vi "load data_backup.vi"(7 "Append dataset":bool, 10 "existing file numbers":string[](array[string]), 11 "existing data cluster":cluster{"array type (2D Dbl)":dbl[][]}[](array[cluster])) -> (2 "data names":string[](array[string]), 3 "data cluster":cluster{"all data":dbl[][]}[](array[cluster]))   [LabVIEW 2020]
uses:
  <vilib>/Utility/file.llb/Read Delimited Spreadsheet (DBL).vi
panel:
  in  "Done":bool
  out "# of importe files":i32
  in  "numbered file":T1={"FILE HEADER"="20120217", "FROM"="012", "TO"="012", "Excluding\nFrom"="", "Excluding\nTo"="", "Start Loading\ndata files"=FALSE, "cancel"=FALSE}
  in  "Cancel button":bool
  in  "Import Menu":T2(ring)
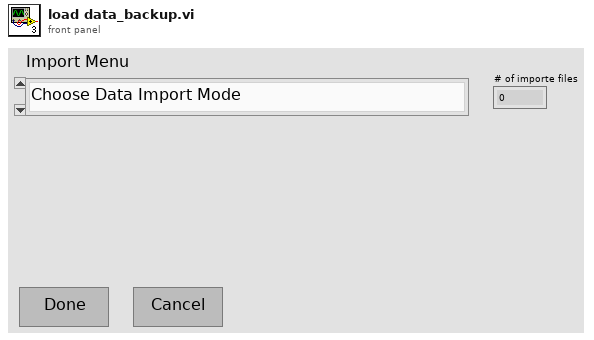
[diagram p1: front panel]
types:
  T1 = cluster{"FILE HEADER":string, "FROM":string, "TO":string, "Excluding\nFrom":string, "Excluding\nTo":string, "Start Loading\ndata files":bool, "cancel":bool}
  T2 = enum16{"Choose Data Import Mode", "Numbered NML Data Acq files saved in the drive", "Import current data being taken", "Manual selection of text file(s) ", "Manual Input of single XY plot(s)", "Manual Input of a worksheet"}
  T3 = enum16{"Choose Data Import Mode", "Numbered NML Data Acq files saved in the drive", "Import current NML Data Acq being taken", "Manual selection of text file(s) ", "Manual Input of XY arrays", "Manual Input of a worksheet"}
  T4 = enum16{"Left Button", "Center Button", "Right Button", "Window Close"}
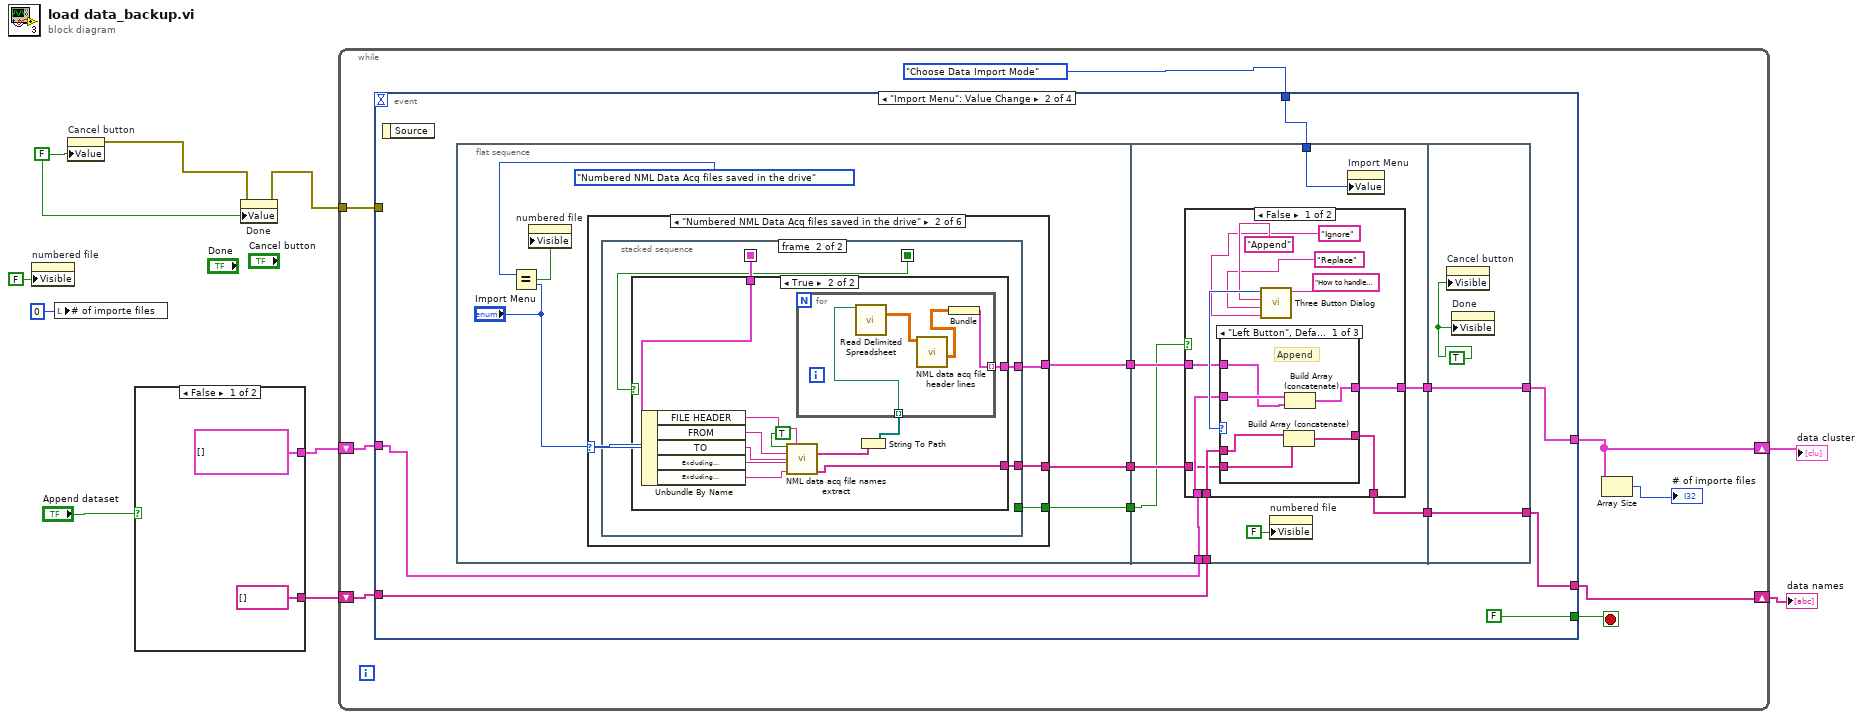
[diagram p0: block diagram]
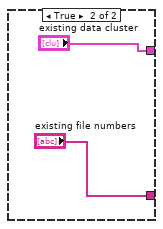
[diagram p2: hidden frame]
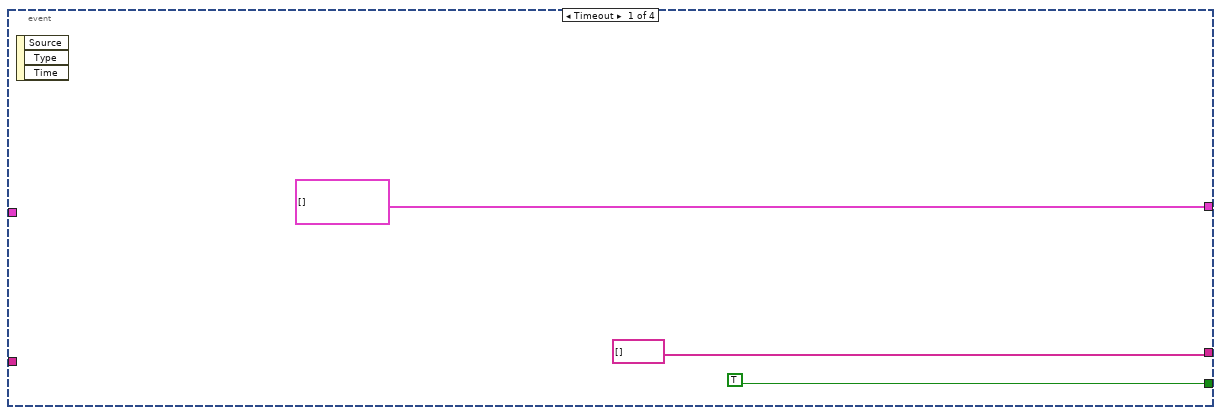
[diagram p3: hidden frame]
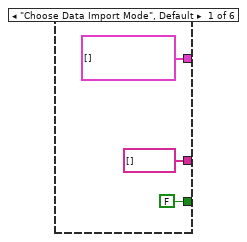
[diagram p4: hidden frame]
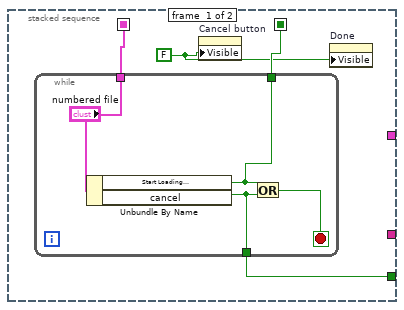
[diagram p5: hidden frame]
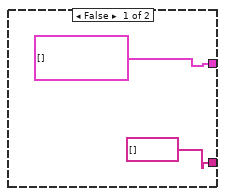
[diagram p6: hidden frame]
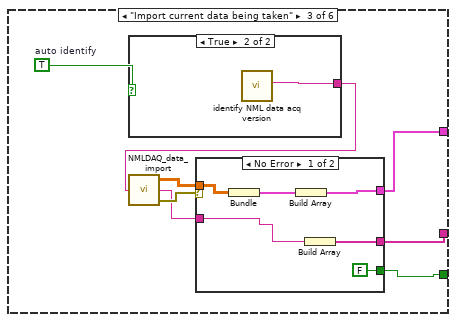
[diagram p7: hidden frame]
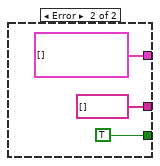
[diagram p8: hidden frame]
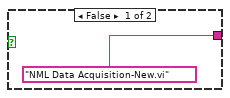
[diagram p9: hidden frame]
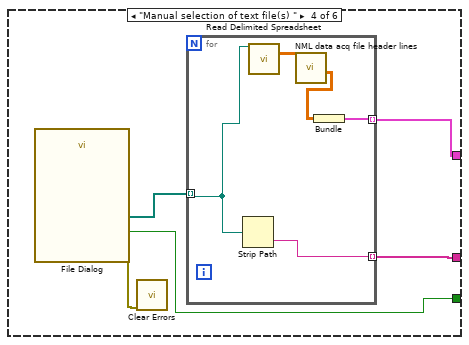
[diagram p10: hidden frame]
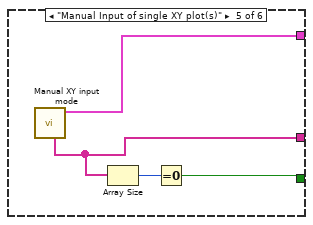
[diagram p11: hidden frame]
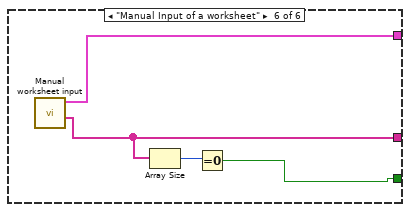
[diagram p12: hidden frame]
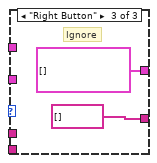
[diagram p14: hidden frame]
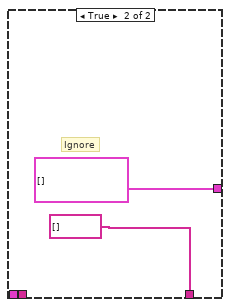
[diagram p15: hidden frame]
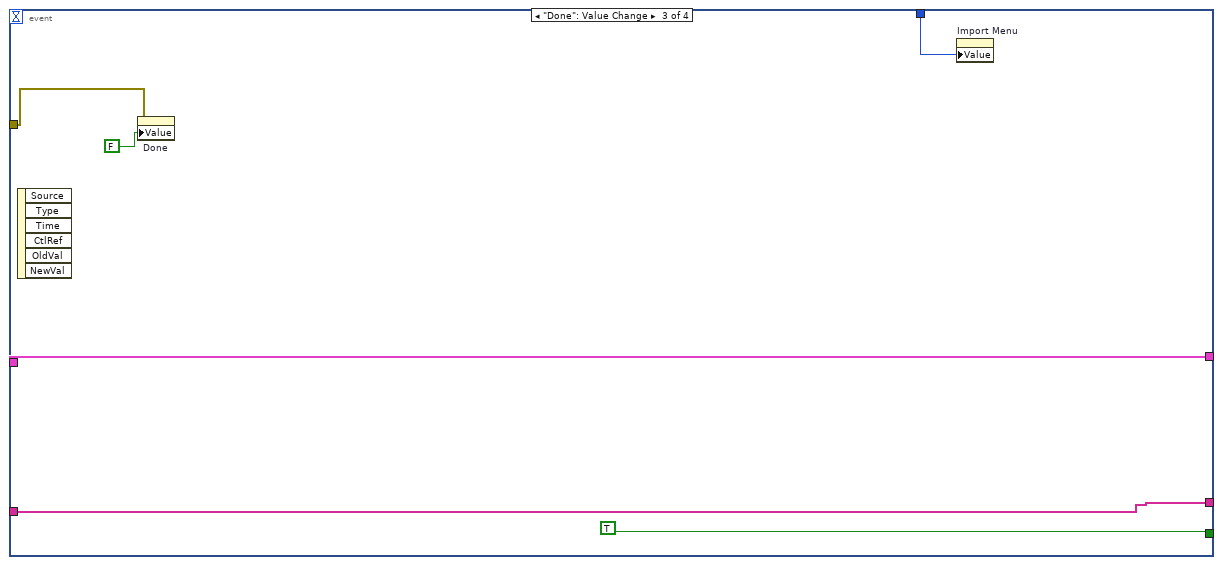
[diagram p16: hidden frame]
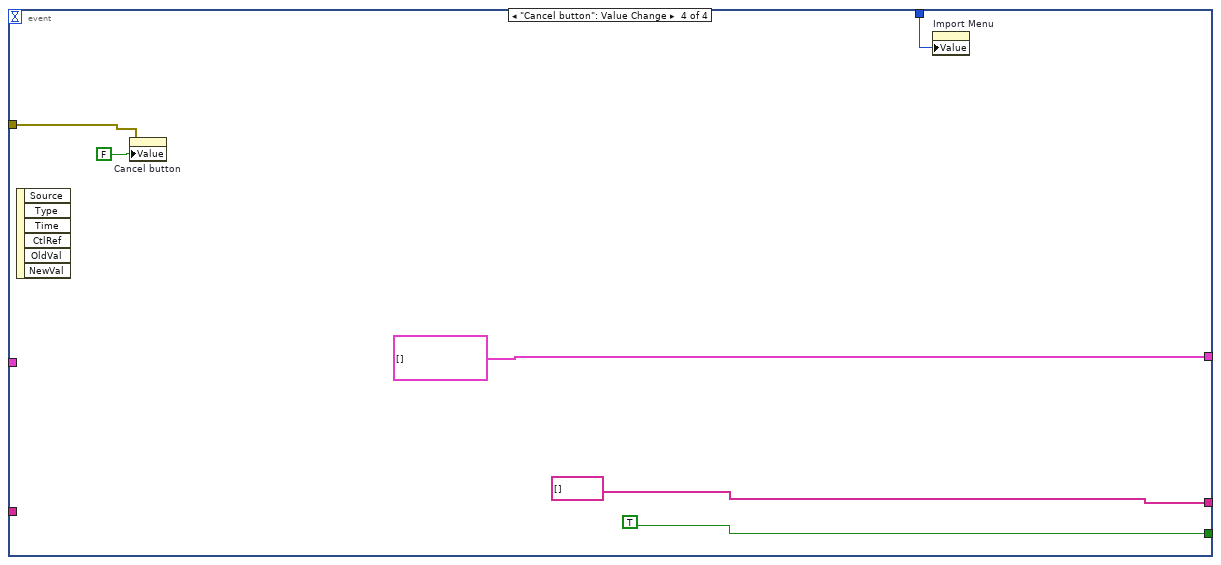
[diagram p17: hidden frame]
diagram:
  w2 = FALSE ("Value (Signaling)")
  n1 = property on="numbered file" class="Clust"("Visible"=FALSE) -> ()  [unwired: 2 in, 2 out]
  n2 = local write "# of importe files"(0 ("# of data files")) -> ()
  n3 = property on="Cancel button" class="Bool (strict)"("Value"=w2) -> (error out=w3:errorcluster)  [unwired: 2 in, 1 out]
  n4 = case shown="False" "Append dataset" {
    tunnel: [cluster{"array type (2D Dbl)":dbl[][]}[] [] ("existing data cluster") "existing data cluster"] -> w6
    tunnel: [string[] [] ("existing file numbers") "existing file numbers"] -> w5
    frame False {
    }
    frame True {
    }
  }
  n5 = property on="Done" class="Bool (strict)"(error in=w3, "Value"=w2) -> (error out=w1:errorcluster)  [unwired: 1 in, 1 out]
  n6 = while {
    shift-right: [w17] -> w7
    shift-left: w6 -> [w21]
    shift-right: [w18] -> w8
    shift-left: w5 -> [w19]
    tunnel: w1 -> [w16]
    stop <- w22 stop-if-true
    n7 = event shown="[1] \"Import Menu\": Value Change" {
      selector: _ -> [_ _ _ _]
      dyn-events: _ -> [_ _ _ _]
      timeout: _ -> [_ _ _ _]
      tunnel: [TRUE FALSE TRUE TRUE] -> w22
      tunnel: [cluster{"array type (2D Dbl)":dbl[][]}[] [] ("Data clusters") w33 w154 cluster{"array type (2D Dbl)":dbl[][]}[] [] ("Data clusters")] -> w17
      tunnel: w21 -> [_ w35 w154 _]
      tunnel: [string[] [] ("file numbers") w32 w153 string[] [] ("file numbers")] -> w18
      tunnel: w19 -> [_ w34 w153 _]
      tunnel: w16 -> [_ _ w152 w158]
      tunnel: T2."Choose Data Import Mode" ("Import Menu") -> [_ w31 w150 w156]
      event Timeout {
        n8 = event-data() -> ()  [unwired: 1 in, 3 out]
      }
      event "Import Menu": Value Change {
        n9 = event-data() -> ()  [unwired: 1 in, 1 out]
        n10 = flat-sequence {
          tunnel: [w40] -> w30
          tunnel: [w39] -> w29
          tunnel: [w37] -> w26
          tunnel: w30 -> [w120]
          tunnel: w29 -> [w121]
          tunnel: w35 -> [w123]
          tunnel: w34 -> [w122]
          tunnel: w31 -> [w116]
          tunnel: [w119] -> w28
          tunnel: [w118] -> w27
          tunnel: w26 -> [w115]
          tunnel: [w148] -> w32
          tunnel: [w149] -> w33
          tunnel: w28 -> [w149]
          tunnel: w27 -> [w148]
          frame #0 {
            n11 = Equal?(x=T3."Numbered NML Data Acq files saved in the drive", y="Import Menu") -> (x = y?=w38:bool)
            n12 = property on="numbered file" class="Clust"("Visible"=w38) -> ()  [unwired: 2 in, 2 out]
            n13 = case shown="\"Numbered NML Data Acq files saved in the drive\"" "Import Menu" {
              tunnel: [cluster{"array type (2D Dbl)":dbl[][]}[] [] ("Data clusters") w48 w79 w101 w110 w114] -> w40
              tunnel: [string[] [] ("file numbers") w47 w80 w99 w109 w113] -> w39
              tunnel: [FALSE ("cancel") w46 w78 w97 w107 w111] -> w37
              frame "Choose Data Import Mode", Default {
              }
              frame "Numbered NML Data Acq files saved in the drive" {
                n14 = stacked-sequence {
                  seq-local: [w52 _] -> [_ w59]
                  seq-local: [w51 _] -> [_ w57]
                  tunnel: [_ w60] -> w48
                  tunnel: [_ w58] -> w47
                  tunnel: [w49 _] -> w46
                  frame #0 {
                    w50 = FALSE ("Visible")
                    n15 = while {
                      tunnel: ["numbered file"] -> w52
                      tunnel: [w54] -> w51
                      tunnel: [w53] -> w49
                      stop <- w55 stop-if-true
                      n16 = Unbundle By Name("numbered file") -> ("Start Loading\ndata files"=w54:bool, "cancel"=w53:bool)
                      n17 = Or(x=w54, y=w53) -> (x .or. y?=w55:bool)
                    }
                    n18 = property on="Cancel button" class="Bool (strict)"("Visible"=w50) -> ()  [unwired: 2 in, 2 out]
                    n19 = property on="Done" class="Bool (strict)"("Visible"=w50) -> ()  [unwired: 2 in, 2 out]
                  }
                  frame #1 {
                    n20 = case shown="True" w57 {
                      tunnel: [cluster{"array type (2D Dbl)":dbl[][]}[] [] ("Data clusters") w72] -> w60
                      tunnel: w59 -> [_ w69]
                      tunnel: [string[] [] ("file numbers") w63] -> w58
                      frame False {
                      }
                      frame True {
                        n21 = Unbundle By Name(w69) -> ("FILE HEADER"=w68:string, "FROM"=w67:string, "TO"=w66:string, "Excluding\nFrom"=w65:string, "Excluding\nTo"=w64:string)
                        n22 = call "NML data acq file names extract.vi"("assign directory"=TRUE, "File name header"=w68, "From"=w67, "To"=w66, "Excluding From"=w65, "Excluding To"=w64) -> ("file paths"=w70:string[], "existing files"=w63:string[])  [unwired: 6 in, 2 out]
                        n23 = String To Path(string=w70) -> (path=w73:path[])
                        n24 = for {
                          tunnel: w73 -> [w76] mode=indexing
                          tunnel: [w77] -> w72 mode=indexing
                          n25 = call-poly <vilib>:"Read Delimited Spreadsheet.vi"("file path (dialog if empty)"=w76) -> ("all rows"=w75:dbl[][])  [unwired: 9 in, 5 out]
                          n26 = call "NML data acq file header lines.vi"("all rows"=w75) -> ("real data?"=w74:dbl[][])  [unwired: 8 in, 2 out]
                          n27 = Bundle("real data?"=w74) -> (w77:cluster{"real data?":dbl[][]})  [unwired: 1 in]
                        }
                      }
                    }
                  }
                }
              }
              frame "Import current data being taken" {
                w84 = TRUE  # auto identify
                n28 = case shown="True" w84 {
                  tunnel: ["NML Data Acquisition-New.vi" ("NML Data Acquisition VI") w96] -> w85
                  frame False {
                  }
                  frame True {
                    n29 = call "identify NML data acq version.vi"() -> ("NML data in the memory"=w96:string)  [unwired: 11 in]
                  }
                }
                n30 = call "NMLDAQ_data_import.vi"("NML Data Acquisition VI"=w85) -> ("data"=w82:dbl[][], "file name"=w81:string, "error out"=w83:errorcluster)
                n31 = case shown="No Error" w83 {
                  tunnel: w82 -> [w90 _]
                  tunnel: w81 -> [w87 _]
                  tunnel: [w89 string[] []] -> w80
                  tunnel: [w88 cluster{"data":dbl[][]}[] []] -> w79
                  tunnel: [FALSE TRUE] -> w78
                  frame No Error {
                    n32 = Bundle("data"=w90) -> (w91:cluster{"data":dbl[][]})  [unwired: 1 in]
                    n33 = Build Array(w91) -> (w88:cluster{"data":dbl[][]}[])
                    n34 = Build Array(w87) -> (w89:string[])
                  }
                  frame Error {
                  }
                }
              }
              frame "Manual selection of text file(s) " {
                n35 = call "File Dialog"() -> ("selected paths"=w100:path[], "cancelled"=w97:bool, "error out"=w98:errorcluster)  [unwired: 12 in, 1 out]
                n36 = call <vilib>:"Clear Errors.vi"("error in (no error)"=w98) -> ()  [unwired: 5 in, 2 out]
                n37 = for {
                  tunnel: w100 -> [w105] mode=indexing
                  tunnel: [w106] -> w101 mode=indexing
                  tunnel: [w104] -> w99 mode=indexing
                  n38 = Strip Path(path=w105) -> (name=w104:string)  [unwired: 1 out]
                  n39 = call-poly <vilib>:"Read Delimited Spreadsheet.vi"("file path (dialog if empty)"=w105) -> ("all rows"=w103:dbl[][])  [unwired: 9 in, 5 out]
                  n40 = call "NML data acq file header lines.vi"("all rows"=w103) -> ("real data?"=w102:dbl[][])  [unwired: 8 in, 2 out]
                  n41 = Bundle("real data?"=w102) -> (w106:cluster{"real data?":dbl[][]})  [unwired: 1 in]
                }
              }
              frame "Manual Input of single XY plot(s)" {
                n42 = call "Manual XY input mode.vi"() -> ("Data clusters"=w110:cluster{"array type (2D Dbl)":dbl[][]}[], "data names"=w109:string[])  [unwired: 7 in, 3 out]
                n43 = Array Size(array=w109) -> (size(s)=w108:i32)
                n44 = Equal To 0?(x=w108) -> (x = 0?=w107:bool)
              }
              frame "Manual Input of a worksheet" {
                n45 = call "Manual worksheet input.vi"() -> ("data names"=w113:string[], "Data clusters"=w114:cluster{"array type (2D Dbl)":dbl[][]}[])  [unwired: 8 in, 2 out]
                n46 = Array Size(array=w113) -> (size(s)=w112:i32)
                n47 = Equal To 0?(x=w112) -> (x = 0?=w111:bool)
              }
            }
          }
          frame #1 {
            n48 = case shown="False" w115 {
              tunnel: w123 -> [w129 _]
              tunnel: w122 -> [w128 _]
              tunnel: w121 -> [w127 _]
              tunnel: w120 -> [w126 _]
              tunnel: [w125 cluster{"array type (2D Dbl)":dbl[][]}[] []] -> w119
              tunnel: [w124 string[] []] -> w118
              frame False {
                n49 = call <vilib>:"Three Button Dialog.vi"("Right Button Text (\"Cancel\")"="Ignore" ("Right Button Text (\"Cancel\")"), "Center Button Text (\"No\")"="Replace" ("Center Button Text (\"No\")"), "Left Button Text (\"Yes\")"="Append" ("Left Button Text (\"Yes\")"), "message"="How to handle the imported data?") -> ("Which Button?"=w134:T4)  [unwired: 7 in]
                n50 = case shown="\"Left Button\", Default" w134 {
                  tunnel: [w140 w142 cluster{"array type (2D Dbl)":dbl[][]}[] []] -> w125
                  tunnel: [w139 w141 string[] []] -> w124
                  tunnel: w129 -> [w138 _ _]
                  tunnel: w128 -> [w137 _ _]
                  tunnel: w127 -> [w136 w141 _]
                  tunnel: w126 -> [w135 w142 _]
                  frame "Left Button", Default {
                    # "Append"
                    n51 = Build Array (concatenate)(w137, w136) -> (w139:string[])
                    n52 = Build Array (concatenate)(w138, w135) -> (w140:cluster{"array type (2D Dbl)":dbl[][]}[])
                  }
                  frame "Center Button" {
                    # "Replace"
                  }
                  frame "Right Button" {
                    # "Ignore"
                  }
                }
              }
              frame True {
                # "Ignore"
              }
            }
            n53 = property on="numbered file" class="Clust"("Visible"=FALSE) -> ()  [unwired: 2 in, 2 out]
            n54 = property on="Import Menu" class="Enum (strict)"("Value"=w116) -> ()  [unwired: 2 in, 2 out]
          }
          frame #2 {
            w147 = TRUE ("Visible")
            n55 = property on="Cancel button" class="Bool (strict)"("Visible"=w147) -> ()  [unwired: 2 in, 2 out]
            n56 = property on="Done" class="Bool (strict)"("Visible"=w147) -> ()  [unwired: 2 in, 2 out]
          }
        }
      }
      event "Done": Value Change {
        n57 = event-data() -> ()  [unwired: 1 in, 6 out]
        n58 = property on="Done" class="Bool (strict)"(error in=w152, "Value"=FALSE ("Value (Signaling)")) -> ()  [unwired: 1 in, 2 out]
        n59 = property on="Import Menu" class="Enum (strict)"("Value"=w150) -> ()  [unwired: 2 in, 2 out]
      }
      event "Cancel button": Value Change {
        n60 = event-data() -> ()  [unwired: 1 in, 6 out]
        n61 = property on="Cancel button" class="Bool (strict)"(error in=w158, "Value"=FALSE ("Value (Signaling)")) -> ()  [unwired: 1 in, 2 out]
        n62 = property on="Import Menu" class="Enum (strict)"("Value"=w156) -> ()  [unwired: 2 in, 2 out]
      }
    }
    n63 = Array Size(array=w17) -> (size(s)=→"# of importe files":i32)
  }
  "data cluster" <- w7
  "data names" <- w8
